vi "dg535 error handler.vi"(2 "error in":errorcluster, 3 "check bit #":dbl min=0.0 max=6.0, 4 "command string":string, 5 "VISA resource name":refnum<visa-resource-name>) -> (0 "error out":errorcluster, 1 "error found":bool)   [LabVIEW 2009]
doc: "This support subVI queries the instrument's error status bits which reports an execution error .\n ERROR FOUND is set to TRUE when an out of range parameter or a delay linkage error causes an execution error . \n This subVI is used in the function subVIs after setting some or all of the instrument's functions .\n The status of ERROR FOUND is then used in the function subVIs to report an error for the parameter that caused it ."
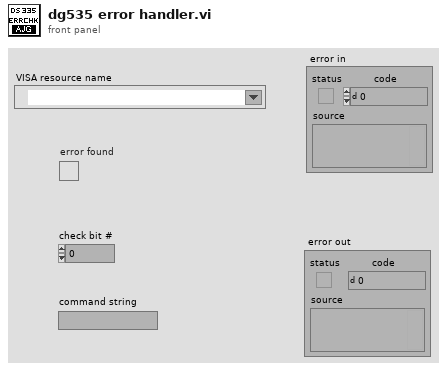
[diagram p1: front panel]
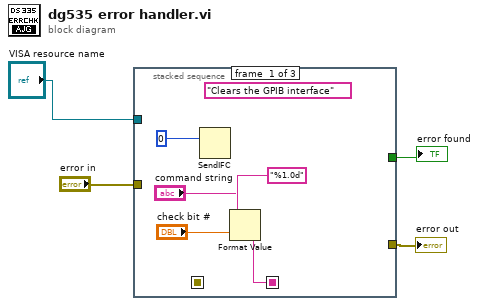
[diagram p0: block diagram]
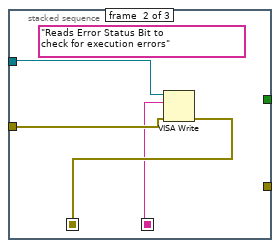
[diagram p2: hidden frame]
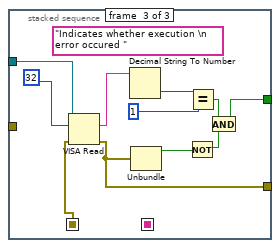
[diagram p3: hidden frame]
diagram:
  n1 = stacked-sequence {
    seq-local: [_ w12 _] -> [_ _ w18]
    seq-local: [w7 _ _] -> [_ w11 _]
    tunnel: "VISA resource name" -> [_ w10 w14]
    tunnel: "error in" -> [_ w13 _]
    tunnel: [_ _ w16] -> w3
    tunnel: [_ _ w19] -> w2
    frame #0 {
      (unwired) "Clears the GPIB interface"
      n2 = SendIFC(3:0) -> ()  [unwired: 1 in, 2 out]
      n3 = Format Value(string ("")="command string", format string="%1.0d", value (0)="check bit #") -> (output string=w7:string)
    }
    frame #1 {
      (unwired) "Reads Error Status Bit to                                                    check for execution errors"
      n4 = VISA Write(VISA resource name=w10, write buffer=w11, error in (no error)=w13) -> (error out=w12:errorcluster)  [unwired: 2 out]
    }
    frame #2 {
      (unwired) "Indicates whether execution \n          error occured "
      n5 = VISA Read(VISA resource name=w14, byte count=32, error in (no error)=w18) -> (read buffer=w15:string, error out=w16:errorcluster)  [unwired: 2 out]
      n6 = Decimal String To Number(string=w15) -> (number=w24:i32)  [unwired: 3 out]
      n7 = Unbundle(w16) -> ("status"=w22:bool)  [unwired: 2 out]
      n8 = Not(x=w22) -> (.not. x?=w21:bool)
      n9 = Equal?(x=w24, y=1) -> (x = y?=w20:bool)
      n10 = And(x=w20, y=w21) -> (x .and. y?=w19:bool)
    }
  }
  "error out" <- w3
  "error found" <- w2
